vi "simulate-robot.vi"() -> ()   [LabVIEW 2019]
uses:
  Robot Global Data.vi
  <vilib>/Rock Robotics/WPI/ThirdParty/JAS_Junk/TrajLib/Trajectory_Library.lvlib
  ROBOT_PICTURE.ctl
  <vilib>/Rock Robotics/WPI/Camera/WPI_CameraImageSize.ctl
panel:
  in  "Finish":bool
  in  "Enable Vision":bool
  in  "Image Size":T1=enum."320x240"
  out "ROBOT":T2
  out "BALL":bool=TRUE
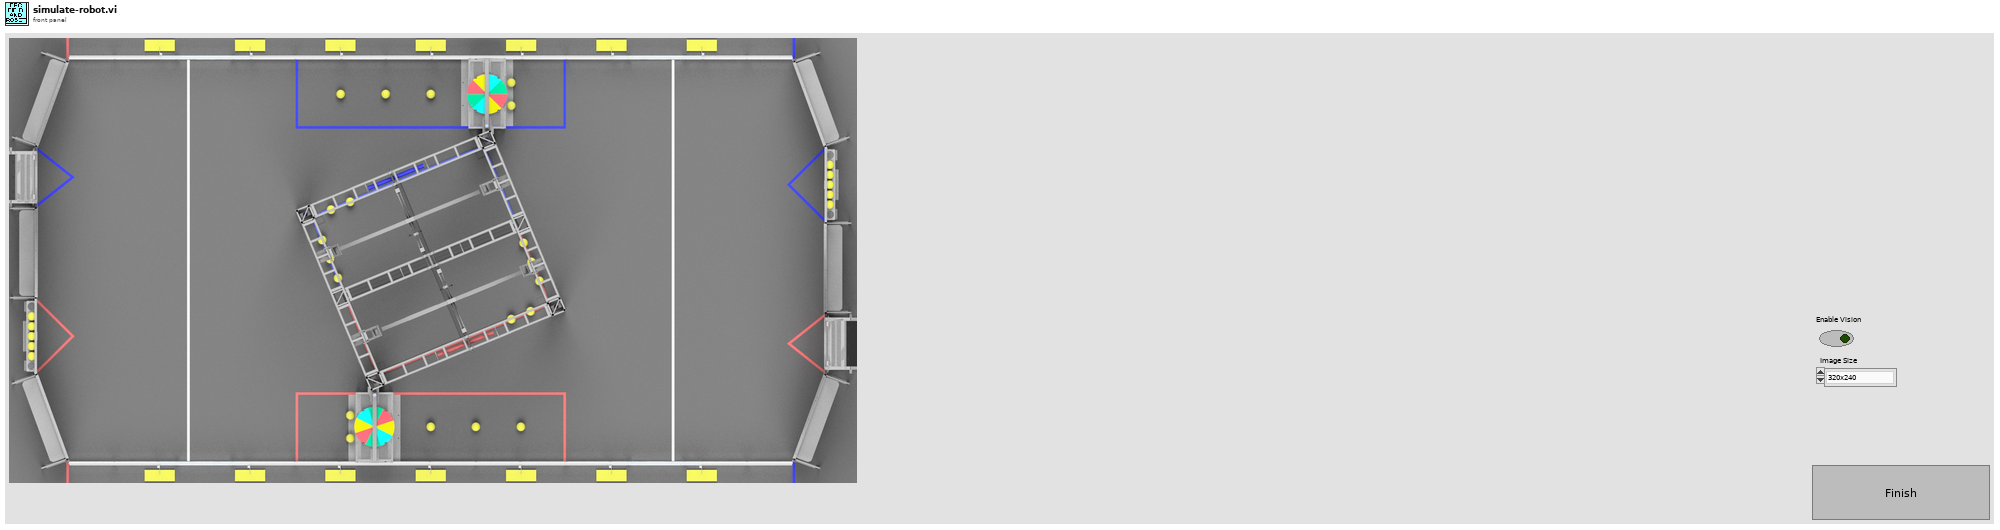
[diagram p1: front panel]
types:
  T1 = typedef "WPI_CameraImageSize.ctl" = enum16{"640x480", "320x240", "160x120", "Custom"}
  T2 = typedef "ROBOT_PICTURE.ctl" = picture
  T3 = typedef "WPI_DriverStationMatch Info.ctl" = cluster{"Autonomous Elapsed Seconds":dbl, "TeleOp Elapsed Seconds":dbl, "Disabled Elapsed Seconds":dbl, "Visited Autonomous":bool, "Visited TeleOp":bool, "Visited Disabled":bool, "Autonomous Settings":cluster{"Autonomous Style":enum16{"Iterative", "Independent"}, "VI Refnum":refnum<vi>}}
  T4 = typedef "WPI_DriverStationDerivedRobotMode.ctl" = enum16{"Init", "Execute", "Stop"}
  T5 = typedef "WPI_DriverStationRobotMode2.ctl" = enum16{"Autonomous Disabled", "Autonomous Enabled", "Teleop Disabled", "Teleop Enabled", "Disconnected", "Finish", "Test Disabled", "Test Enabled", "Emergency Stopped"}
  T6 = typedef "Rotated_Picture_TypeDef.ctl" = cluster{"ONE-8-bit pixmap":u8[][], "Two-Array":cdb[][], "Three-Numeric":i32, "Four-Numeric":i32, "Five-Numeric":cdb, "Six-colors":u32[], "Seven-new element/subarray":u32, "Eight-Cluster":cluster{"[0]":i32, "[1]":i32}}
  T7 = typedef "Trajectory_Library.lvlib/SWERVE_DRIVE_ODOMETRY.ctl" = cluster{"POSE":T8, "GyroOffset":T10, "PreviousAngle":T10, "PrevModulePositions":T11[], "NumModules":i32}
  T8 = typedef "Trajectory_Library.lvlib/POSE2D.ctl" = cluster{"TRANSLATION":T9, "ROTATION":T10}
  T9 = typedef "Trajectory_Library.lvlib/TRANSLATION2D.ctl" = cluster{"X":dbl, "Y":dbl}
  T10 = typedef "Trajectory_Library.lvlib/ROTATION2D.ctl" = cluster{"VALUE":dbl, "COS":dbl, "SIN":dbl}
  T11 = typedef "Trajectory_Library.lvlib/SWERVE_DRIVE_MODULE_POSITION.ctl" = cluster{"Distance":dbl, "Angle":T10, "P":bool}
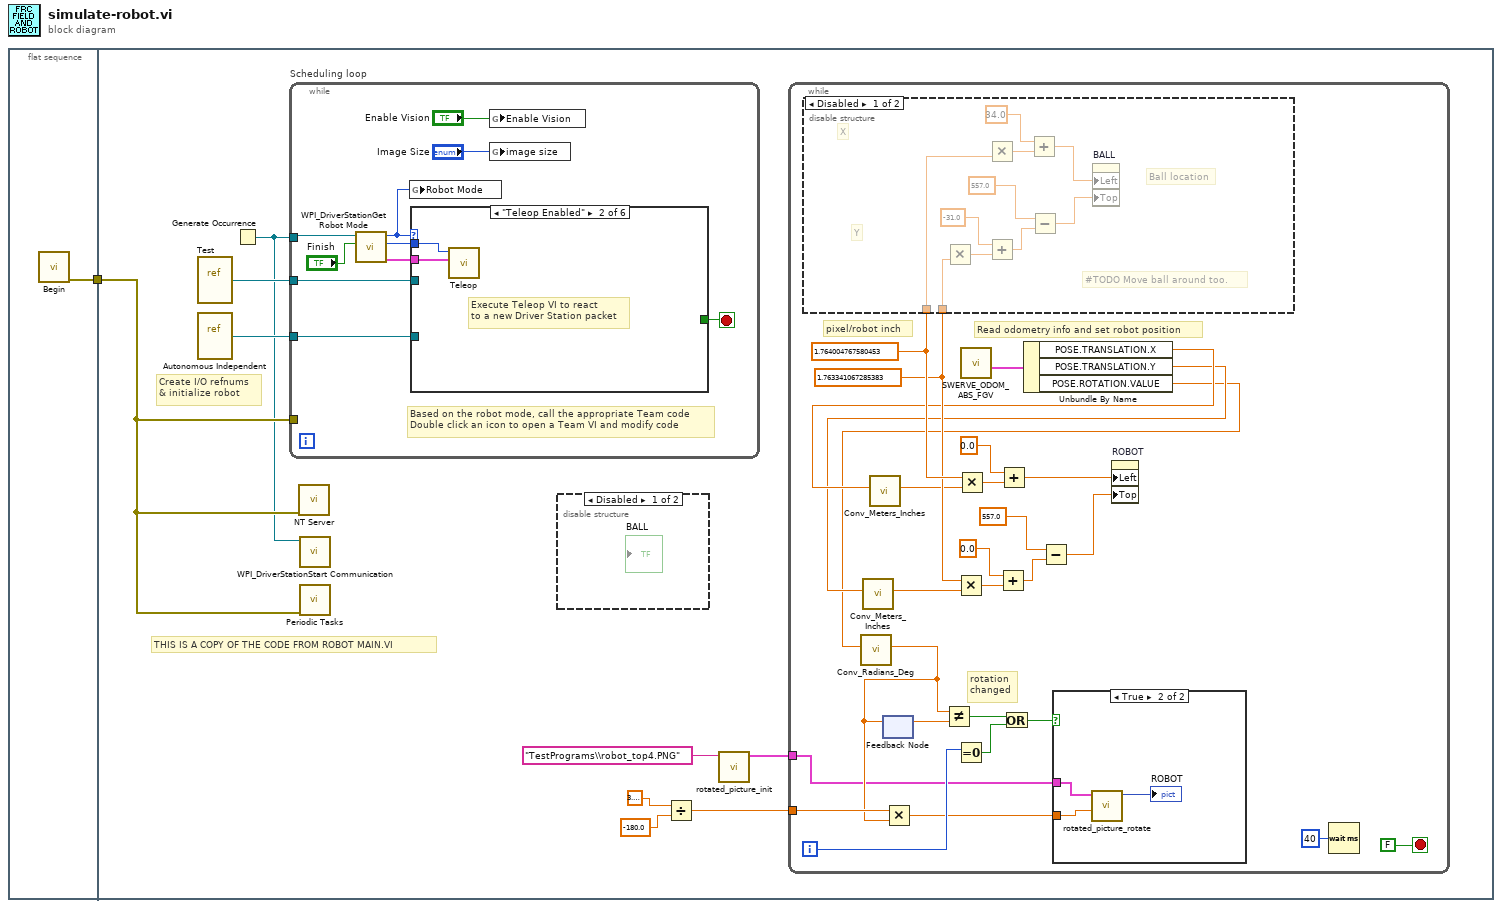
[diagram p0: block diagram]
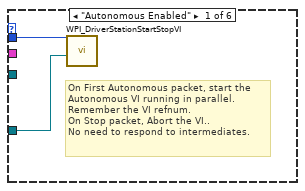
[diagram p3: hidden frame]
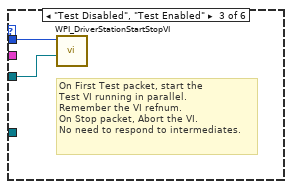
[diagram p4: hidden frame]
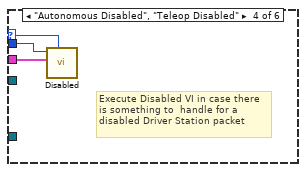
[diagram p5: hidden frame]
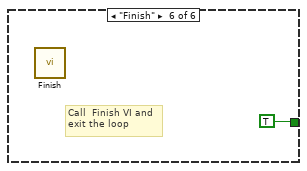
[diagram p7: hidden frame]
diagram:
  n1 = flat-sequence {
    tunnel: [w2] -> w1
    tunnel: w1 -> [w6]
    frame #0 {
      n2 = call "Begin.vi"() -> ("error out"=w2:errorcluster)  [unwired: 11 in]
    }
    frame #1 {
      # "THIS IS A COPY OF THE CODE FROM ROBOT MAIN.VI"
      # "Create I/O refnums\n& initialize robot"
      n3 = vi-ref "Test.vi"() -> (w7:refnum<vi>)
      n4 = vi-ref "Autonomous Independent.vi"() -> (w8:refnum<vi>)
      n5 = Generate Occurrence() -> (w5:refnum<k4>)
      n6 = while "Scheduling loop" {
        tunnel: w5 -> [w20]
        tunnel: w6 -> [_]
        tunnel: w8 -> [w15]
        tunnel: w7 -> [w13]
        stop <- w17 stop-if-true
        # "Based on the robot mode, call the appropriate Team code\nDouble click an icon to open a Team VI and modify code"
        n7 = call <vilib>:"WPI_DriverStationGet Robot Mode.vi"("Finish"="Finish", "DS Occurrence"=w20) -> ("Match Info out"=w18:T3, "Call Context"=w21:T4, "Robot Mode"=w12:T5)  [unwired: 7 out]
        n8 = global write "Robot Global Data.vi" "Robot Mode"(w12) -> ()
        n9 = case shown="\"Teleop Enabled\"" w12 {
          selector: w12 -> [_ _ _ w28 _ _]
          tunnel: w21 -> [w23 w25 w27 w30 _ _]
          tunnel: w18 -> [_ w24 _ w29 _ _]
          tunnel: [_ _ _ _ _ TRUE] -> w17
          tunnel: w15 -> [w22 _ _ _ _ _]
          tunnel: w13 -> [_ _ w26 _ _ _]
          frame "Autonomous Enabled" {
            # "On First Autonomous packet, start the\nAutonomous VI running in parallel.\nRemember the VI refnum.\nOn Stop packet, Abort the VI..\nNo need to respond to intermediates."
            n10 = call <vilib>:"WPI_DriverStationStartStopVI.vi"("VI in"=w22, "Call Context"=w23) -> ()  [unwired: 10 in]
          }
          frame "Teleop Enabled" {
            # "Execute Teleop VI to react\nto a new Driver Station packet"
            n11 = call "Teleop.vi"("Match Info"=w24, "Call Context"=w25) -> ()  [unwired: 1 in, 9 out]
          }
          frame "Test Disabled", "Test Enabled" {
            # "On First Test packet, start the\nTest VI running in parallel.\nRemember the VI refnum.\nOn Stop packet, Abort the VI.\nNo need to respond to intermediates."
            n12 = call <vilib>:"WPI_DriverStationStartStopVI.vi"("VI in"=w26, "Call Context"=w27) -> ()  [unwired: 10 in]
          }
          frame "Autonomous Disabled", "Teleop Disabled" {
            # "Execute Disabled VI in case there\nis something to  handle for a\ndisabled Driver Station packet"
            n13 = call "Disabled.vi"("Robot Mode"=w28, "Match Info"=w29, "Call Context"=w30) -> ()  [unwired: 1 in, 8 out]
          }
          frame "Disconnected", Default {
            # "Driver Station packet didn't arrive.\nPossibly useful for diagnostics"
          }
          frame "Finish" {
            # "Call  Finish VI and\nexit the loop"
            n14 = call "Finish.vi"() -> ()  [unwired: 1 in, 7 out]
          }
        }
        n15 = global write "Robot Global Data.vi" "Enable Vision"("Enable Vision") -> ()
        n16 = global write "Robot Global Data.vi" "image size"("Image Size") -> ()
      }
      n17 = call <vilib>:"NT Server.vi"("error in (no error)"=w6) -> ()  [unwired: 11 in]
      n18 = call <vilib>:"WPI_DriverStationStart Communication.vi"("occurrence"=w5) -> ()  [unwired: 2 in, 9 out]
      n19 = call "Periodic Tasks.vi"("error in"=w6) -> ()  [unwired: 11 in]
      n20 = disable-structure shown="Disabled" {
        frame Disabled {
        }
        frame Enabled {
        }
      }
      n21 = Divide(x=3.141592653589793, y=-180.0 ("value")) -> (x/y=w11:dbl)
      n22 = call "rotated_picture_init.vi"("Picture FIle Name"="TestPrograms\\robot_top4.PNG" ("name or relative path")) -> ("RotatedPictureInfo"=w3:T6)  [unwired: 10 in]
      n23 = while {
        tunnel: w11 -> [w58]
        tunnel: w3 -> [w32]
        i -> [w41]
        stop <- FALSE stop-if-true
        w45 = 1.763341067285383
        w46 = 1.764004767580453
        # "Read odometry info and set robot position"
        # "pixel/robot inch"
        # "rotation\nchanged"
        n24 = disable-structure shown="Disabled" {
          disable-tunnel: w46 -> [w68 _]
          disable-tunnel: w45 -> [w61 _]
          frame Disabled {
            # "#TODO Move ball around too."
            # "Y"
            # "X"
            # "Ball location"
            n25 = Multiply(y=w61) -> (x=w59:dbl, x*y=w66:dbl)
            n26 = Multiply(y=w68) -> (x=w60:dbl, x*y=w70:dbl)
            n27 = Add(x=-31.0, y=w66) -> (x+y=w63:dbl)
            n28 = Add(x=34.0, y=w70) -> (x+y=w67:dbl)
            n29 = Subtract(x=557.0, y=w63) -> (x-y=w62:dbl)
            n30 = property on="BALL" class="Bool (strict)"("Left"=w67, "Top"=w62) -> ()  [unwired: 2 in, 2 out]
          }
          frame Enabled {
          }
        }
        n31 = feedback #1() -> (w55:dbl)  [unwired: 1 in]
        n32 = Equal To 0?(x=w41) -> (x = 0?=w42:bool)
        n33 = call "SWERVE_ODOM_ABS_FGV.vi"() -> ("out SWERVE_DRIVE_ODOMETRY"=w40:T7)  [unwired: 11 in]
        n34 = Unbundle By Name(w40) -> ("POSE.TRANSLATION.X"=w38:dbl, "POSE.TRANSLATION.Y"=w36:dbl, "POSE.ROTATION.VALUE"=w34:dbl)
        n35 = call <vilib>:"Conv_Radians_Deg.vi"("Radians"=w34) -> ("Degrees"=w35:dbl)  [unwired: 10 in]
        n36 = call <vilib>:"Conv_Meters_Inches.vi"("Meters"=w36) -> ("Inches"=w37:dbl)  [unwired: 10 in]
        n37 = call <vilib>:"Conv_Meters_Inches.vi"("Meters"=w38) -> ("Inches"=w39:dbl)  [unwired: 10 in]
        n38 = feedback-in #1(w35) -> ()
        n39 = Multiply(x=w58, y=w35) -> (x*y=w33:dbl)
        n40 = Not Equal?(x=w35, y=w55) -> (x != y?=w43:bool)
        n41 = Multiply(x=w45, y=w37) -> (x*y=w52:dbl)
        n42 = Multiply(x=w46, y=w39) -> (x*y=w54:dbl)
        n43 = Add(x=0.0, y=w52) -> (x+y=w48:dbl)
        n44 = Add(x=0.0, y=w54) -> (x+y=w49:dbl)
        n45 = Or(x=w43, y=w42) -> (x .or. y?=w44:bool)
        n46 = Subtract(x=557.0, y=w48) -> (x-y=w47:dbl)
        n47 = case shown="True" w44 {
          tunnel: w33 -> [_ w71]
          tunnel: w32 -> [_ w72]
          frame False {
          }
          frame True {
            n48 = call "rotated_picture_rotate.vi"("Angle"=w71, "RotatedPictureInfo"=w72) -> ("new picture"=→"ROBOT":picture)  [unwired: 9 in]
          }
        }
        n49 = property on="ROBOT" class="Pict (strict)"("Left"=w49, "Top"=w47) -> ()  [unwired: 2 in, 2 out]
        n50 = Wait (ms)(milliseconds to wait=u32 40) -> ()  [unwired: 1 out]
      }
    }
  }
